vi "Update Embedded Progress Bar Indicator.vi"(8 "Error In":errorcluster, 10 "Progress Bar Event":T1, 11 "Progress Bar Refnum":refnum<vi>) -> (0 "Error Out":errorcluster, 3 "Quit?":bool)   [LabVIEW 2021, in "GUI.lvlib"]
uses:
  Embedded Progress Bar Q Element.ctl
  GUI.lvlib
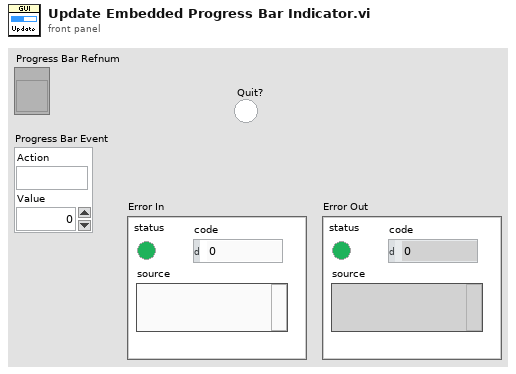
[diagram p1: front panel]
types:
  T1 = typedef "GUI.lvlib/Embedded Progress Bar Q Element.ctl" = cluster{"Action":string, "Value":dbl}
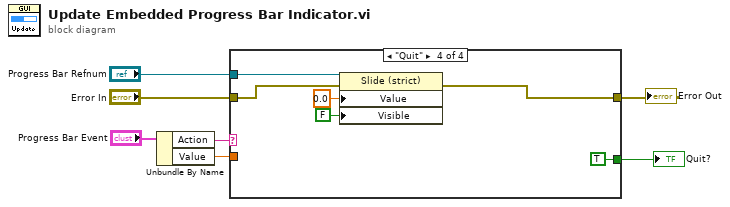
[diagram p0: block diagram]
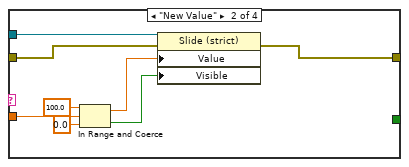
[diagram p3: hidden frame]
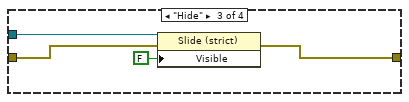
[diagram p4: hidden frame]
diagram:
  n1 = Unbundle By Name("Progress Bar Event") -> ("Action"=w4:string, "Value"=w6:dbl)
  n2 = case shown="\"Quit\"" w4 {
    tunnel: [_ _ _ TRUE] -> w5
    tunnel: w6 -> [_ w16 _ _]
    tunnel: "Progress Bar Refnum" -> [_ w13 w20 w25]
    tunnel: "Error In" -> [w8 w10 w18 w22]
    tunnel: [w8 w9 w17 w21] -> w1
    frame "", Default {
    }
    frame "New Value" {
      n3 = In Range and Coerce(upper limit=100.0, x=w16, lower limit=0.0) -> (coerced(x)=w12:dbl, In Range?=w11:bool)
      n4 = property class="Slide (strict)"(reference=w13, error in=w10, "Value"=w12, "Visible"=w11) -> (error out=w9:errorcluster)  [unwired: 1 out]
    }
    frame "Hide" {
      n5 = property class="Slide (strict)"(reference=w20, error in=w18, "Visible"=FALSE) -> (error out=w17:errorcluster)  [unwired: 1 out]
    }
    frame "Quit" {
      n6 = property class="Slide (strict)"(reference=w25, error in=w22, "Value"=0.0, "Visible"=FALSE) -> (error out=w21:errorcluster)  [unwired: 1 out]
    }
  }
  "Quit?" <- w5
  "Error Out" <- w1
